vi "Read Text Differences.vi"(8 "error in":errorcluster, 11 "Diff File Path":path) -> (0 "error out":errorcluster, 2 "Removed":i32, 3 "Added":i32)   [LabVIEW 2020, in "Peer Review.lvclass"]
uses:
  Peer Review.lvclass
  Peer Review.lvclass/Peer Review.ctl
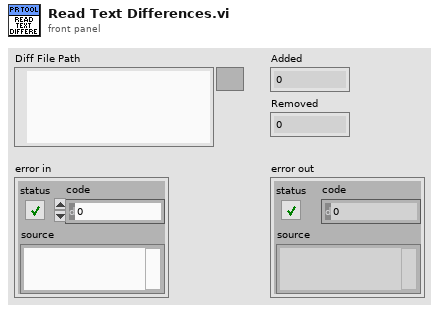
[diagram p1: front panel]
types:
  T1 = enum16{"open", "replace", "create", "open or create", "replace or create", "replace or create with confirmation"}
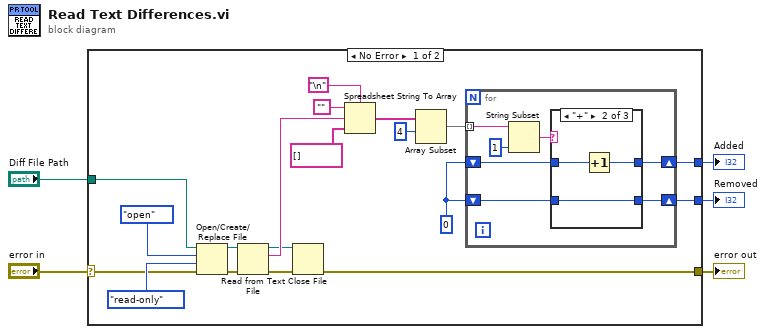
[diagram p0: block diagram]
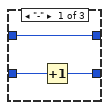
[diagram p2: hidden frame]
diagram:
  n1 = case shown="No Error" "error in" {
    selector: "error in" -> [w10 w40]
    tunnel: [w8 w40] -> w4
    tunnel: "Diff File Path" -> [w9 _]
    tunnel: [w7 _] -> w2
    tunnel: [w6 _] -> w1
    frame No Error {
      w16 = 0
      n2 = Open/Create/Replace File(file path (use dialog)=w9, error in=w10, operation (0:open)=T1."open", access (0:read/write)=enum16{"read/write", "read-only", "write-only"}."read-only") -> (refnum out=w18:refnum<file>, error out=w19:errorcluster)  [unwired: 2 in, 1 out]
      n3 = Read from Text File(file (use dialog)=w18, error in=w19) -> (refnum out=w21:refnum<file>, text=w22:string, error out=w20:errorcluster)  [unwired: 2 in, 1 out]
      n4 = Close File(refnum=w21, error in=w20) -> (error out=w8:errorcluster)  [unwired: 1 out]
      n5 = Spreadsheet String To Array(delimiter (Tab)="\n", format string="", spreadsheet string=w22, array type (2D Dbl)=string[] []) -> (array=w24:string[])
      n6 = Array Subset(array=w24, index=4) -> (w23:string[])  [unwired: 1 in]
      n7 = for {
        tunnel: w23 -> [w31] mode=indexing
        shift-right: [w28] -> w6
        shift-left: w16 -> [w27]
        shift-right: [w26] -> w7
        shift-left: w16 -> [w25]
        n8 = String Subset(string=w31, length (rest)=1 ("length (rest)")) -> (substring=w29:string)  [unwired: 1 in]
        n9 = case shown="\"+\"" w29 {
          tunnel: [w32 w37 w39] -> w28
          tunnel: w27 -> [w33 w37 w39]
          tunnel: [w34 w35 w38] -> w26
          tunnel: w25 -> [w34 w36 w38]
          frame "-" {
            n10 = Increment(x=w33) -> (x+1=w32:i32)
          }
          frame "+" {
            n11 = Increment(x=w36) -> (x+1=w35:i32)
          }
          frame Default {
          }
        }
      }
    }
    frame Error {
    }
  }
  "error out" <- w4
  "Removed" <- w1
  "Added" <- w2
